vi "Exercise 1.vi"() -> ()   [LabVIEW 2012]
panel:
  in  "Numeric 2":dbl
  out "Boolean":bool
  in  "Numeric":dbl
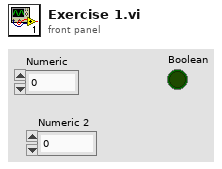
[diagram p1: front panel]
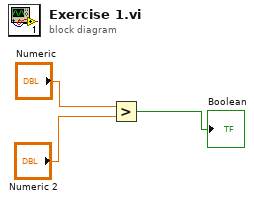
[diagram p0: block diagram]
diagram:
  n1 = Greater?(x="Numeric", y="Numeric 2") -> (0:→"Boolean":bool)
